vi "Get_Inlet_temps_from_files.vi"(5 "Templated Plotted channels":string[][](array[string]), 7 "Templated Channel Names":string[](array[string]), 8 "Last File":bool, 9 "First file":bool, 10 "Filename":path, 11 "Selected Rows":i32[](array[numeric])) -> ()   [LabVIEW 2014]
uses:
  Globals/Constants_global.vi
  Results_plotter_Global.vi
  <vilib>/gmath/interp.llb/Interpolate 2D Scattered (1D).vi
  <vilib>/gmath/NI_AAL_Interpolation.lvlib
panel:
  out "Array 2":dbl[](array[numeric])
  out "Y Axis Current":dbl[](array[numeric])
  out "Array":dbl[](array[numeric])
  in  "Z Location":u16(ring) items=["X (mm)::", "Z (mm)::", "Y:Thermistor:(mm)", "T::", "U::", "U/Uref::", "Uref::", "Inst::", "File::", "EnFlo_Tunnel:Trav3 Pos:Y", "RV (T):Y Position:Y (mm)", "Multi Run:Start Time:", "Tref::", "Multi Run:Row:Number", "T-Tref::", "Seconds:since:1st Jan", "Flow:Measurement:Time", "Inlet:Offset:Temperature"]
  in  "Y Location":u16(ring) items=["X (mm)::", "Z (mm)::", "Y:Thermistor:(mm)", "T::", "U::", "U/Uref::", "Uref::", "Inst::", "File::", "EnFlo_Tunnel:Trav3 Pos:Y", "RV (T):Y Position:Y (mm)", "Multi Run:Start Time:", "Tref::", "Multi Run:Row:Number", "T-Tref::", "Seconds:since:1st Jan", "Flow:Measurement:Time", "Inlet:Offset:Temperature"]
  out "Ch names Out":string[](array[string])
  out "Channel Values Out":string[][](array[string])
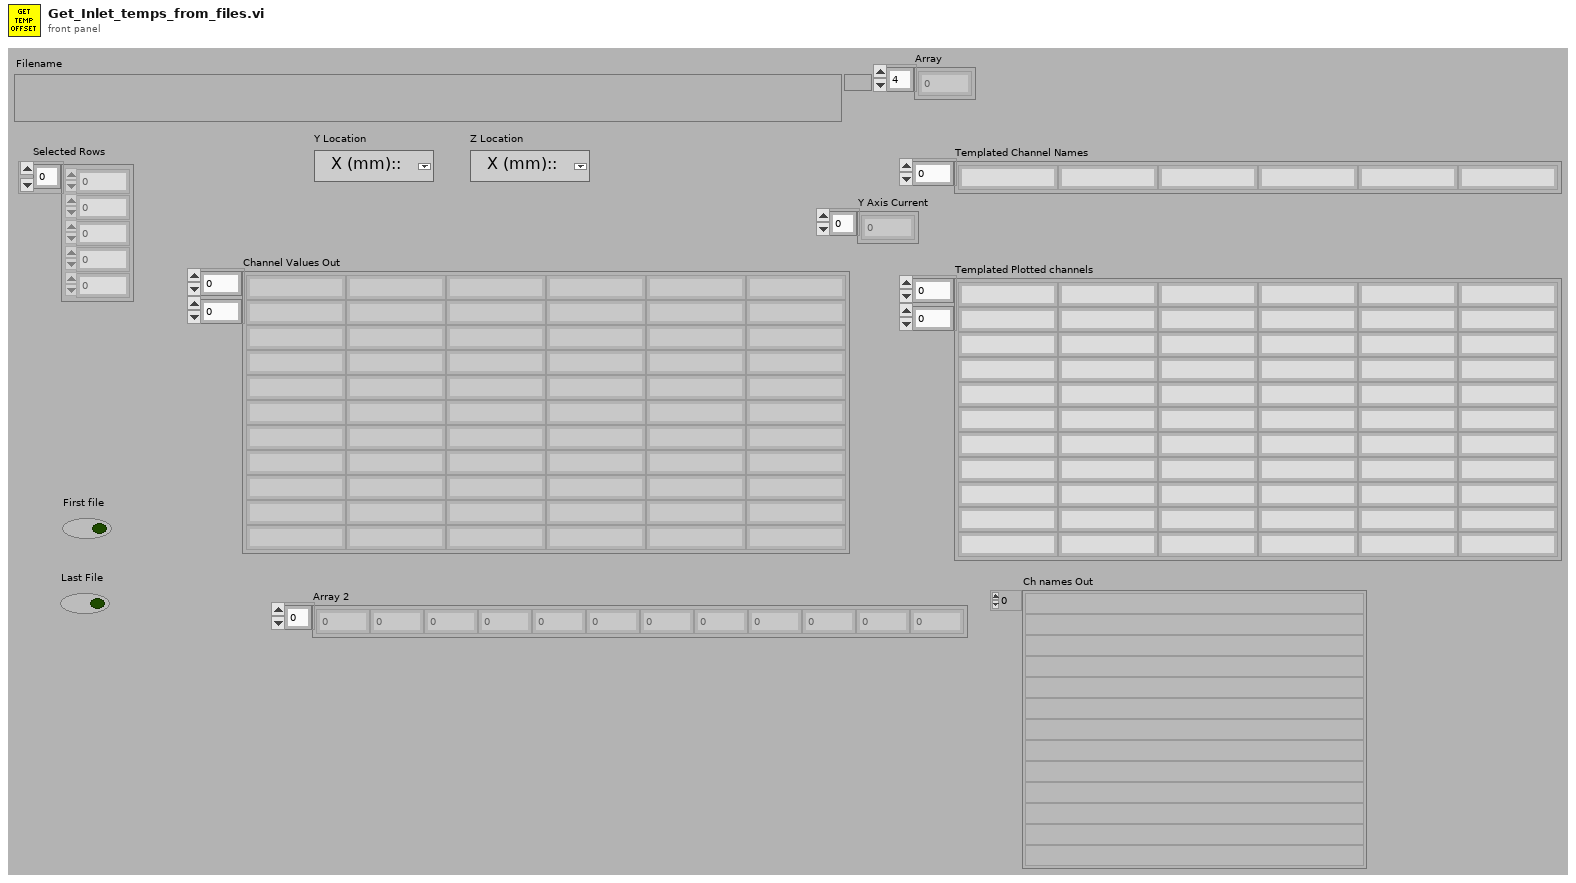
[diagram p1: front panel]
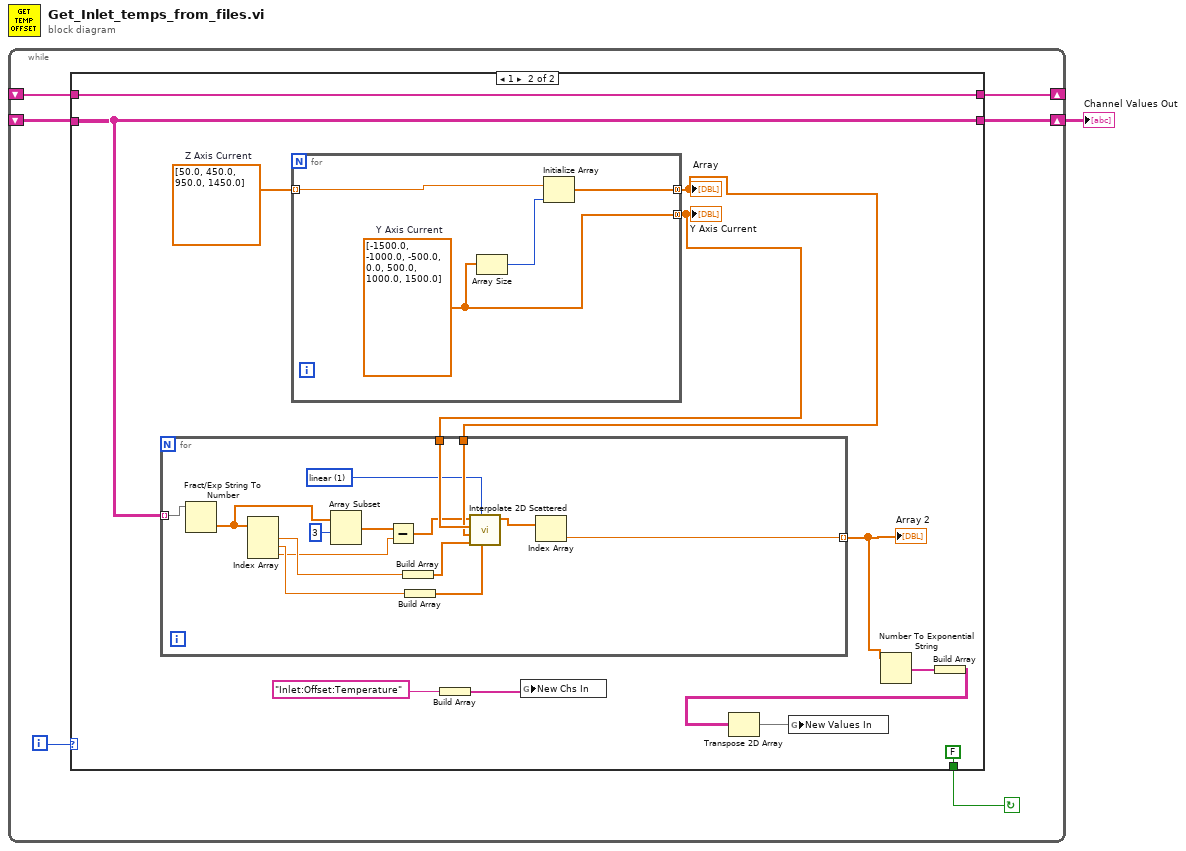
[diagram p0: block diagram]
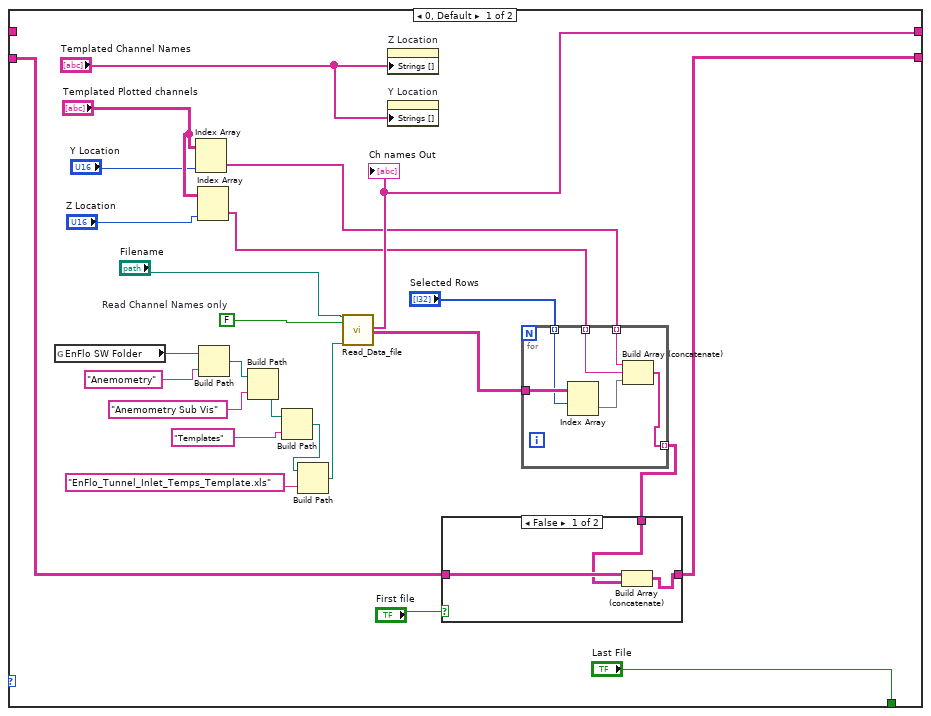
[diagram p2: hidden frame]
diagram:
  n1 = while {
    shift-right: [w6] -> w1
    shift-left: _ -> [w7]
    shift-right: [w4] -> _
    shift-left: _ -> [w3]
    i -> [w2]
    stop <- w5 continue-if-true
    n2 = case shown="1" w2 {
      tunnel: [w25 w52] -> w6
      tunnel: w7 -> [w24 w52]
      tunnel: ["Last File" FALSE ("Last File")] -> w5
      tunnel: [w22 w54] -> w4
      tunnel: w3 -> [_ w54]
      frame 0, Default {
        w29 = FALSE  # Read Channel Names only
        n3 = global read "Constants_global.vi" "EnFlo SW Folder"() -> (w20:path)
        n4 = Index Array(array="Templated Plotted channels", index (col)="Y Location") -> (element=w9:string[])  [unwired: 1 in]
        n5 = Index Array(array="Templated Plotted channels", index (col)="Z Location") -> (element=w8:string[])  [unwired: 1 in]
        n6 = Build Path(base path=w20, name or relative path="Anemometry") -> (appended path=w18:path)
        n7 = Build Path(base path=w18, name or relative path="Anemometry Sub Vis") -> (appended path=w15:path)
        n8 = Build Path(base path=w15, name or relative path="Templates") -> (appended path=w16:path)
        n9 = Build Path(base path=w16, name or relative path="EnFlo_Tunnel_Inlet_Temps_Template.xls") -> (appended path=w31:path)
        n10 = call "Read_Data_file.vi"("Results file"="Filename", "Read Channel Names only"=w29, "Template File"=w31) -> ("Ch names Out"=w22:string[], "Channel Values Out"=w32:string[][])  [unwired: 2 in, 13 out]
        "Ch names Out" <- w22
        n11 = property on="Z Location" class="Ring (strict)"("Strings []"="Templated Channel Names") -> ()  [unwired: 2 in, 2 out]
        n12 = property on="Y Location" class="Ring (strict)"("Strings []"="Templated Channel Names") -> ()  [unwired: 2 in, 2 out]
        n13 = for {
          tunnel: w32 -> [w42]
          tunnel: "Selected Rows" -> [w41] mode=indexing
          tunnel: [w37] -> w26 mode=indexing
          tunnel: w9 -> [w39] mode=indexing
          tunnel: w8 -> [w38] mode=indexing
          n14 = Index Array(array=w42, index (row)=w41) -> (element=w40:string[])  [unwired: 1 in]
          n15 = Build Array (concatenate)(w39, w38, w40) -> (w37:string[])
        }
        n16 = case shown="False" "First file" {
          tunnel: [w33 w36] -> w25
          tunnel: w26 -> [w34 w36]
          tunnel: w24 -> [w35 _]
          frame False {
            n17 = Build Array (concatenate)(w35, w34) -> (w33:string[][])
          }
          frame True {
          }
        }
      }
      frame 1 {
        w51 = dbl[] [50.0, 450.0, 950.0, 1450.0]  # Z Axis Current
        n18 = for {
          tunnel: [w58] -> w50 mode=concatenating
          tunnel: w51 -> [w56] mode=indexing
          tunnel: [w55] -> w49 mode=concatenating
          w58 = dbl[] [-1500.0, -1000.0, -500.0, 0.0, 500.0, 1000.0, 1500.0]  # Y Axis Current
          n19 = Array Size(array=w58) -> (size(s)=w57:i32)
          n20 = Initialize Array(w56, w57) -> (w55:dbl[])
        }
        "Array" <- w49
        "Y Axis Current" <- w50
        n21 = for {
          tunnel: w52 -> [w73] mode=indexing
          tunnel: w50 -> [w70]
          tunnel: w49 -> [w69]
          tunnel: [w63] -> w46 mode=indexing
          w62 = 1 items=["nearest", "linear", "cubic", "biharmonic spline "] ("method")
          n22 = Fract/Exp String To Number(string=w73) -> (number=w72:dbl[])  [unwired: 3 in, 1 out]
          n23 = Index Array(array=w72) -> (element #1=w68:dbl, element #2=w66:dbl, element #3=w60:dbl)  [unwired: 3 in]
          n24 = Array Subset(array=w72, index=3) -> (w61:dbl[])  [unwired: 1 in]
          n25 = Subtract(x=w61, y=w60) -> (x-y=w59:dbl[])
          n26 = Build Array(w68) -> (w67:dbl[])
          n27 = Build Array(w66) -> (w65:dbl[])
          n28 = call-poly <vilib>:"Interpolate 2D Scattered.vi"("Yi"=w65, "method"=w62, "Xi"=w67, "Y"=w69, "X"=w70, "Z"=w59) -> ("Zi"=w64:dbl[])  [unwired: 4 in, 1 out]
          n29 = Index Array(array=w64) -> (element=w63:dbl)  [unwired: 1 in]
        }
        "Array 2" <- w46
        n30 = Build Array("Inlet:Offset:Temperature") -> (w47:string[])
        n31 = global write "Results_plotter_Global.vi" "New Chs In"(w47) -> ()
        n32 = Number To Exponential String(number=w46) -> (E-format string=w45:string[])  [unwired: 3 in]
        n33 = Build Array(w45) -> (w44:string[][])
        n34 = Transpose 2D Array(2D array=w44) -> (transposed array=w43:string[][])
        n35 = global write "Results_plotter_Global.vi" "New Values In"(w43) -> ()
      }
    }
  }
  "Channel Values Out" <- w1
